vi "Build.vi"(7 "bulid type":T1, 8 "error in (no error)":errorcluster, 9 "save build info to solution":bool=TRUE, 11 "package builder solution path":path) -> (0 "error out":errorcluster, 3 "command line standard output":string)   [LabVIEW 2021, in "NI Package Builder API.lvlib"]
uses:
  NI Package Builder API.lvlib
  build type.ctl
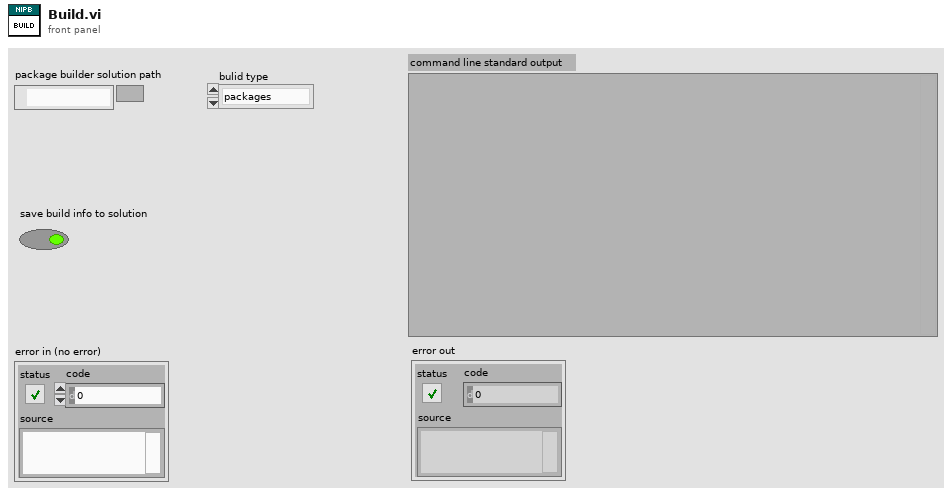
[diagram p1: front panel]
types:
  T1 = typedef "NI Package Builder API.lvlib/build type.ctl" = enum16{"packages", "feeds", "solution"}
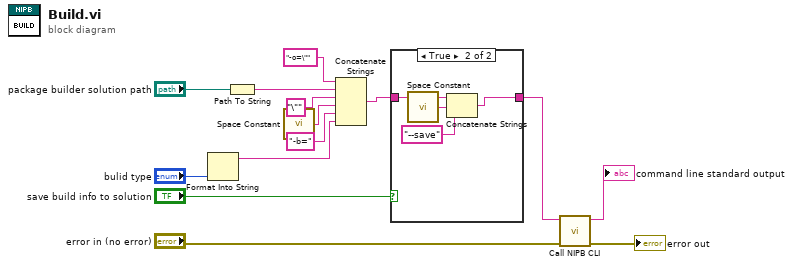
[diagram p0: block diagram]
diagram:
  n1 = Format Into String("bulid type") -> (resulting string=w7:string)  [unwired: 3 in, 1 out]
  n2 = Path To String(path="package builder solution path") -> (string=w10:string)
  n3 = call <vilib>:"Space Constant.vi"() -> ("String"=w3:string)
  n4 = Concatenate Strings("-o=\"" ("string"), w10, "\"", w3, "-b=" ("string"), w7) -> (w6:string)
  n5 = case shown="True" "save build info to solution" {
    tunnel: w6 -> [w15 w19]
    tunnel: [w15 w16] -> w4
    frame False {
    }
    frame True {
      n6 = call <vilib>:"Space Constant.vi"() -> ("String"=w18:string)
      n7 = Concatenate Strings(w19, w18, "--save" ("string")) -> (w16:string)
    }
  }
  n8 = call "Call NIPB CLI.vi"("error in (no error)"="error in (no error)", "command"=w4) -> ("error out"=→"error out":errorcluster, "command line standard output"=→"command line standard output":string)  [unwired: 8 in]
